vi "Configure Beeper.vi"(8 "error in (no error)":errorcluster, 9 "beeper mode (0:imm)":u16(ring) items=["immediate beep", "enable beeper functions", "disable beeper functions"], 11 "VISA resource name":refnum<visa-resource-name>) -> (0 "error out":errorcluster, 3 "VISA resource name out":refnum<visa-resource-name>)   [LabVIEW 2016, in "Agilent 4263X.lvlib"]
doc: "This VI configures the instrument's beeper mode."
uses:
  <instrlib>/Agilent 4263X/Agilent 4263X.lvlib
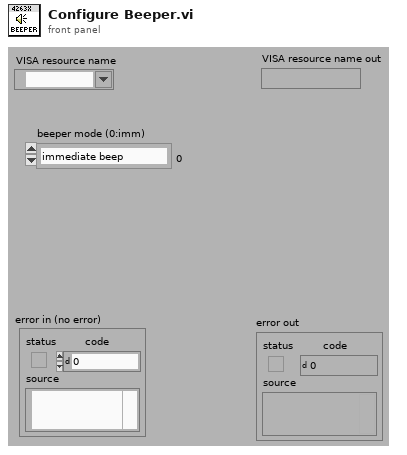
[diagram p1: front panel]
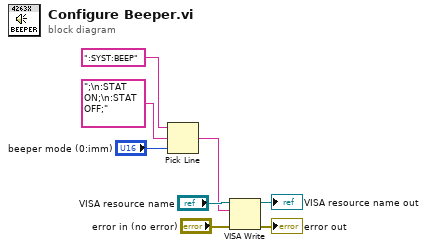
[diagram p0: block diagram]
diagram:
  n1 = Pick Line(string ("")=":SYST:BEEP", multi-line string=";\n:STAT ON;\n:STAT OFF;", line index="beeper mode (0:imm)") -> (output string=w1:string)
  n2 = VISA Write(VISA resource name="VISA resource name", write buffer=w1, error in (no error)="error in (no error)") -> (VISA resource name out=→"VISA resource name out":refnum<visa-resource-name>, error out=→"error out":errorcluster)  [unwired: 1 out]
